vi "visitAllObjects.vi"(0 "HGF_ThreadTask":refnum<class "HGF_ThreadTask.lvclass">, 7 "HGF_Visitor":refnum<class "HGF_Visitor.lvclass">, 11 "error in (no error)":errorcluster) -> (4 "dup HGF_ThreadTask":refnum<class "HGF_ThreadTask.lvclass">, 15 "error out":errorcluster)   [LabVIEW 2014, in "HGF_BaseClasses.lvlib" / "HGF_ThreadTask.lvclass"]
doc: "Viasit all memeber objects"
uses:
  HGF_ThreadTask.lvclass
  HGF_Visitable/HGF_Visitable.lvclass
  HGF_Event/HGF_Event.lvclass
  HGF_Visitor/HGF_Visitor.lvclass
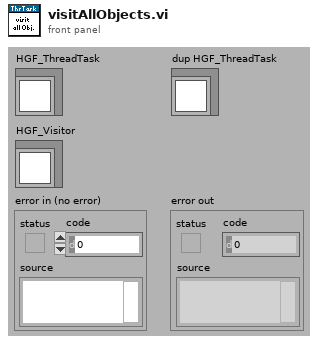
[diagram p1: front panel]
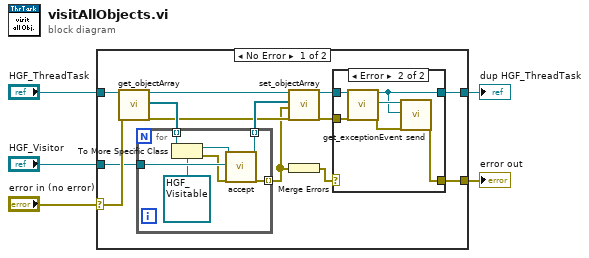
[diagram p0: block diagram]
diagram:
  n1 = case shown="No Error" "error in (no error)" {
    selector: "error in (no error)" -> [w7 w35]
    tunnel: [w8 w35] -> w4
    tunnel: [w9 w34] -> w2
    tunnel: "HGF_ThreadTask" -> [w10 w34]
    tunnel: "HGF_Visitor" -> [w6 _]
    frame No Error {
      n2 = call "get_objectArray.vi"("HGF_ThreadTask"=w10, "error in (no error)"=w7) -> ("dup HGF_ThreadTask"=w18:refnum<class "HGF_ThreadTask.lvclass">, "objectArray"=w17:refnum<class>[], "error out"=w15:errorcluster)  [unwired: 15 out]
      n3 = for {
        tunnel: [w33] -> w14 mode=indexing
        tunnel: w17 -> [w28] mode=indexing
        tunnel: [w32] -> w16 mode=indexing
        tunnel: w6 -> [w31]
        n4 = To More Specific Class(target class=refnum<class "HGF_Visitable.lvclass"> refnum ("HGF_BaseClasses.lvlib:HGF_Visitable.lvclass"), reference=w28) -> (specific class reference=w30:refnum<class "HGF_Visitable.lvclass">, error out=w27:errorcluster)  [unwired: 1 in]
        n5 = call "accept.vi"("HGF_Visitable"=w30, "HGF_Visitor"=w31, "error in (no error)"=w27) -> ("dup HGF_Visitable"=w32:refnum<class "HGF_Visitable.lvclass">, "error out"=w33:errorcluster)  [unwired: 15 out]
      }
      n6 = call "set_objectArray.vi"("HGF_ThreadTask"=w18, "objectArray"=w16, "errorArray"=w14, "error in (no error)"=w15) -> ("dup HGF_ThreadTask"=w13:refnum<class "HGF_ThreadTask.lvclass">, "error out"=w12:errorcluster)  [unwired: 14 out]
      n7 = Merge Errors(w14) -> (w11:errorcluster)
      n8 = case shown="Error" w11 {
        tunnel: w13 -> [w20 w26]
        tunnel: [w20 w21] -> w9
        tunnel: w12 -> [w19 w25]
        tunnel: [w19 w22] -> w8
        frame No Error {
        }
        frame Error {
          n9 = call "get_exceptionEvent.vi"("HGF_ThreadTask"=w26, "error in (no error)"=w25) -> ("dup HGF_ThreadTask"=w21:refnum<class "HGF_ThreadTask.lvclass">, "exceptionEvent"=w24:refnum<class "HGF_Event.lvclass">, "error out"=w23:errorcluster)  [unwired: 15 out]
          n10 = call-dynamic "send.vi"("HGF_Event"=w24, "Object"=w21, "error in (no error)"=w23) -> ("error out"=w22:errorcluster)  [unwired: 2 in, 14 out]
        }
      }
    }
    frame Error {
    }
  }
  "error out" <- w4
  "dup HGF_ThreadTask" <- w2
